vi "SaveDefault.vi"(0 "vi path":path) -> ()   [LabVIEW 2011]
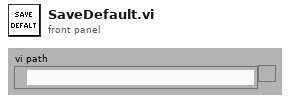
[diagram p1: front panel]
types:
  T1 = enum32{"Invalid", "Standard", "Closed", "Hidden", "Minimized", "Maximized"}
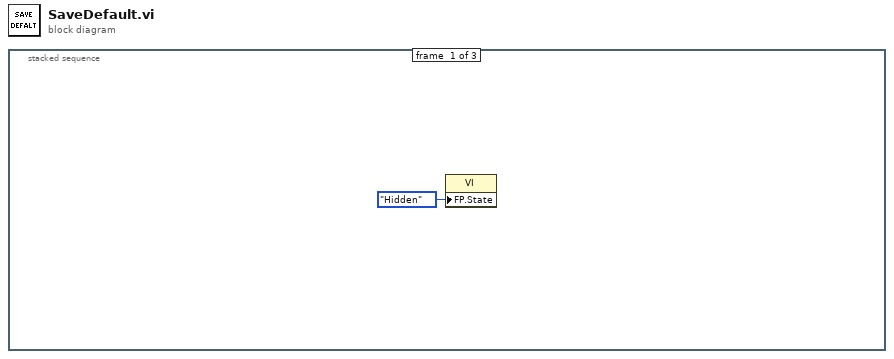
[diagram p0: block diagram]
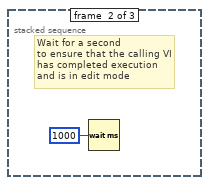
[diagram p2: hidden frame]
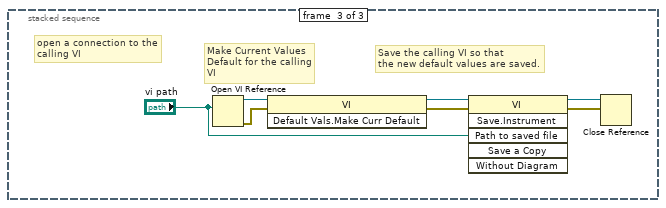
[diagram p3: hidden frame]
diagram:
  n1 = stacked-sequence {
    frame #0 {
      n2 = property class="VI"("FP.State"=T1."Hidden" ("Front Panel Window:State")) -> ()  [unwired: 2 in, 2 out]
    }
    frame #1 {
      # "Wait for a second \nto ensure that the calling VI \nhas completed execution \nand is in edit mode"
      n3 = Wait (ms)(milliseconds to wait=u32 1000) -> ()  [unwired: 1 out]
    }
    frame #2 {
      # "Save the calling VI so that\nthe new default values are saved."
      # "Make Current Values\nDefault for the calling \nVI"
      # "open a connection to the \ncalling VI"
      n4 = Open VI Reference(vi path="vi path") -> (vi reference=w7:refnum<vi>, error out=w6:errorcluster)  [unwired: 5 in]
      n5 = invoke class="VI" method="Default Vals.Make Curr Default"(reference=w7, error in=w6) -> (reference out=w5:refnum<vi>, error out=w4:errorcluster)  [unwired: 1 in, 1 out]
      n6 = invoke class="VI" method="Save.Instrument"(reference=w5, error in=w4, "Path to saved file"="vi path") -> (reference out=w9:refnum<vi>, error out=w8:errorcluster)  [unwired: 3 in, 4 out]
      n7 = Close Reference(reference=w9, error in (no error)=w8) -> ()  [unwired: 1 out]
    }
  }
